vi "InitSequence.vi"(0 "ActXDSO In":refnum<k7>, 2 "Num of Sequences":i32=10, 3 "error in (no error)":errorcluster) -> (5 "ActXDSO Out":refnum<k7>, 8 "error out":errorcluster)   [LabVIEW 2022 SP3]
panel:
  # "Optional"
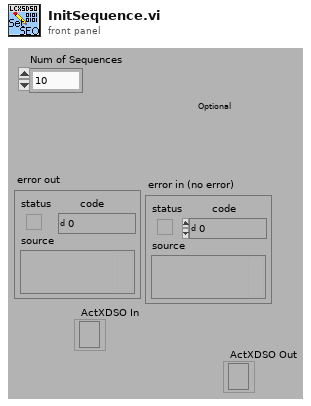
[diagram p1: front panel]
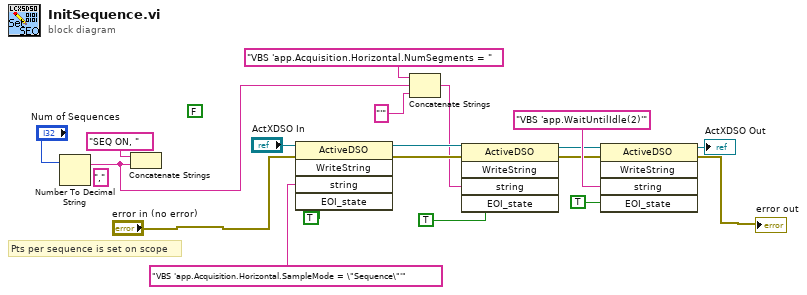
[diagram p0: block diagram]
diagram:
  (unwired) FALSE
  (unwired) ","
  # "Pts per sequence is set on scope"
  n1 = Number To Decimal String(number="Num of Sequences") -> (decimal integer string=w14:string)  [unwired: 1 out]
  n2 = Concatenate Strings("SEQ ON, ", w14) -> ()  [unwired: 1 out]
  n3 = invoke class="ActiveDSO" method="WriteString"(reference="ActXDSO In", error in="error in (no error)", "string"="VBS 'app.Acquisition.Horizontal.SampleMode = \"Sequence\"'", "EOI_state"=TRUE) -> (reference out=w10:refnum<k7>, error out=w11:errorcluster)  [unwired: 1 in, 3 out]
  n4 = Concatenate Strings("VBS 'app.Acquisition.Horizontal.NumSegments = ", w14, "'") -> (w7:string)
  n5 = invoke class="ActiveDSO" method="WriteString"(reference=w10, error in=w11, "string"=w7, "EOI_state"=TRUE) -> (reference out=w4:refnum<k7>, error out=w3:errorcluster)  [unwired: 1 in, 3 out]
  n6 = invoke class="ActiveDSO" method="WriteString"(reference=w4, error in=w3, "string"="VBS 'app.WaitUntilIdle(2)'", "EOI_state"=TRUE) -> (reference out=→"ActXDSO Out":refnum<k7>, error out=→"error out":errorcluster)  [unwired: 1 in, 3 out]
